vi "ma_Pre-process max number of tones.vi"(9 "max #tones":i32=4, 11 "three fingers in":T1[](array[typedef]) {"spectrum" format="%.2f"; "df" format="%.2f"; "f0" format="%.2f"}) -> (2 "number of tones":i32, 3 "three fingers out":T1[](array[typedef]) {"spectrum" format="%.2f"; "df" format="%.2f"; "f0" format="%.2f"})   [LabVIEW 2020, in "NI_MAPro.lvlib"]
uses:
  NI_MAPro.lvlib
  ma_sml_Spectrum Cluster (complex).ctl
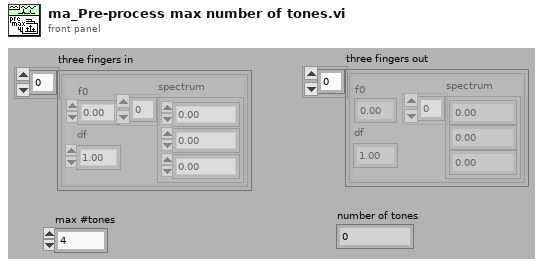
[diagram p1: front panel]
types:
  T1 = typedef "NI_MAPro.lvlib/ma_sml_Spectrum Cluster (complex).ctl" = cluster{"f0":dbl, "df":dbl, "spectrum":cdb[]}
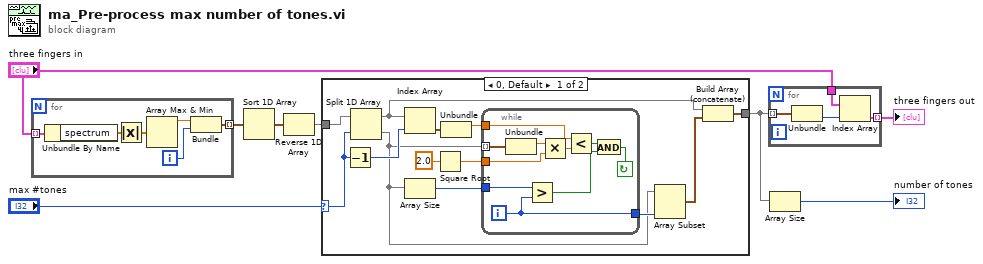
[diagram p0: block diagram]
diagram:
  n1 = for {
    tunnel: "three fingers in" -> [w14] mode=indexing
    tunnel: [w9] -> w8 mode=indexing
    i -> [w10]
    n2 = Unbundle By Name(w14) -> ("spectrum"=w13:cdb[])
    n3 = Absolute Value(x=w13) -> (abs(x)=w12:dbl[])
    n4 = Array Max & Min(array=w12) -> (max value=w11:dbl)  [unwired: 3 out]
    n5 = Bundle(w11, w10) -> (w9:cluster{dbl, i32})  [unwired: 1 out]
  }
  n6 = Sort 1D Array(array=w8) -> (sorted array=w7:cluster{dbl, i32}[])
  n7 = Reverse 1D Array(array=w7) -> (reversed array=w2:cluster{dbl, i32}[])
  n8 = case shown="0, Default" "max #tones" {
    selector: "max #tones" -> [w15 _]
    tunnel: [w21 w38] -> w4
    tunnel: w2 -> [w19 w38]
    frame 0, Default {
      n9 = Decrement(x=w15) -> (x-1=w27:i32)
      n10 = Split 1D Array(array=w19, index=w15) -> (first subarray=w22:cluster{dbl, i32}[], second subarray=w16:cluster{dbl, i32}[])
      n11 = Index Array(array=w22, index=w27) -> (element=w26:cluster{dbl, i32})
      n12 = Array Size(array=w16) -> (size(s)=w20:i32)
      n13 = Square Root(x=2.0) -> (sqrt(x)=w24:dbl)
      n14 = Unbundle(w26) -> (w23:dbl)  [unwired: 1 out]
      n15 = while {
        tunnel: w16 -> [w33] mode=indexing
        tunnel: w24 -> [w36]
        tunnel: w23 -> [w34]
        tunnel: w20 -> [w28]
        tunnel: [w29] -> w18
        i -> [w29]
        stop <- w30 continue-if-true
        n16 = Unbundle(w33) -> (w37:dbl)  [unwired: 1 out]
        n17 = Greater?(x=w28, y=w29) -> (0:w31:bool)
        n18 = Multiply(x=w37, y=w36) -> (x*y=w35:dbl)
        n19 = Less?(x=w34, y=w35) -> (x < y?=w32:bool)
        n20 = And(x=w32, y=w31) -> (x .and. y?=w30:bool)
      }
      n21 = Array Subset(array=w16, length=w18) -> (w17:cluster{dbl, i32}[])  [unwired: 1 in]
      n22 = Build Array (concatenate)(w22, w17) -> (w21:cluster{dbl, i32}[])
    }
    frame ..-1 {
    }
  }
  n23 = for {
    tunnel: w4 -> [w42] mode=indexing
    tunnel: "three fingers in" -> [w40]
    tunnel: [w39] -> w5 mode=indexing
    n24 = Unbundle(w42) -> (w41:i32)  [unwired: 1 out]
    n25 = Index Array(array=w40, index=w41) -> (element=w39:T1)
  }
  "three fingers out" <- w5
  n26 = Array Size(array=w4) -> (size(s)=→"number of tones":i32)
